vi "XIPIN_ICON_(ChipScope_Pro_-_Integrated_Controller)_1_06_a.vi"   [LabVIEW 2017]
doc: "The LogiCORE(TM) IP ChipScope(TM) Pro Integrated CONtroller core (ICON) provides an interface between the JTAG Boundary Scan (BSCAN) interface of the FPGA device and the ChipScope Pro cores.\n------------------------------------\n<b>Need License</b> : No"
uses:
  <vilib>/rvi/XilinxIP/XIPIN_XNode/niFpgaXIPIN.xnode
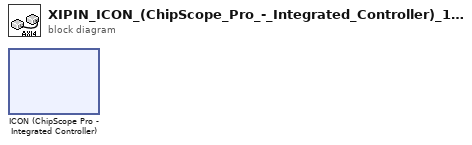
[diagram p0: block diagram]
diagram:
  n1 = xnode ("ICON (ChipScope Pro - Integrated Controller)")() -> ()
